vi "Read Armed.vi"(8 "error in (no error)":errorcluster, 11 "Pulse Recorder in":refnum<class "Pulse Recorder.lvclass">) -> (0 "error out":errorcluster, 2 "Armed":bool, 3 "Pulse Recorder out":refnum<class "Pulse Recorder.lvclass">)   [LabVIEW 2018, in "Pulse Recorder.lvclass"]
uses:
  Pulse Recorder.lvclass
  Pulse Recorder.lvclass/Pulse Recorder.ctl
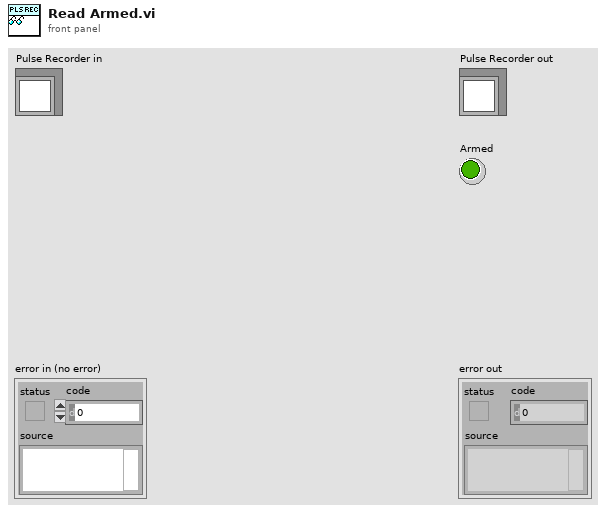
[diagram p1: front panel]
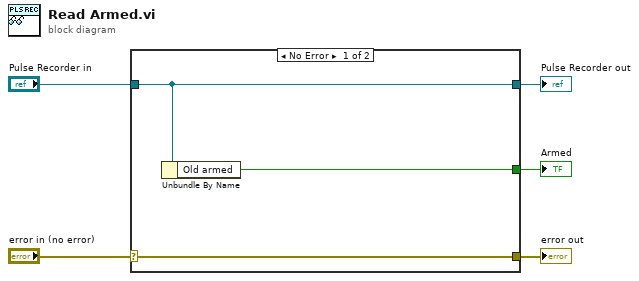
[diagram p0: block diagram]
diagram:
  n1 = case shown="No Error" "error in (no error)" {
    selector: "error in (no error)" -> [w8 w9]
    tunnel: [w8 w9] -> w4
    tunnel: [w7 w10] -> w2
    tunnel: "Pulse Recorder in" -> [w7 w10]
    tunnel: [w6 _] -> w1
    frame No Error {
      n2 = Unbundle By Name(w7) -> ("Old armed"=w6:bool)
    }
    frame Error {
    }
  }
  "error out" <- w4
  "Pulse Recorder out" <- w2
  "Armed" <- w1
